vi "Send-clients-list.vi"(8 "error in (no error)":errorcluster, 9 "Sender ID":i32, 10 "Sender":string, 11 "ModComm in":T1) -> (0 "error out":errorcluster, 3 "ModComm out":T1)   [LabVIEW 2013, in "SLMServer.lvlib" / "SLMServer.lvclass"]
uses:
  SLMServer.lvclass
  Object-reference.ctl
  SA-SLMAPI/Sources/Get-clients/Get-clients.lvclass
  SLMServer.lvclass/SLMServer.ctl
  SA-SLMAPI/Sources/Get-clients/Get-clients.lvclass/Get-clients.ctl
  Read Client IDs.vi
  Read Clients.vi
  SA-SLMAPI/Sources/Get-clients/Write Client IDs.vi
  SA-SLMAPI/Sources/Get-clients/Write Client types.vi
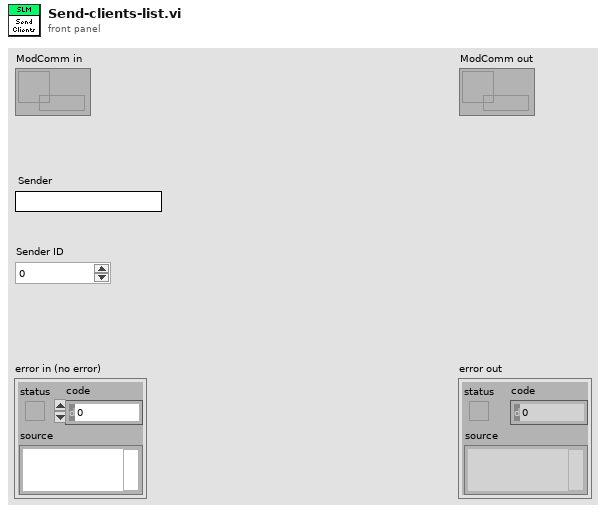
[diagram p1: front panel]
types:
  T1 = typedef "SLMServer.lvlib/SLMServer.lvclass/Object-reference.ctl" = refnum<data-value>
  T2 = typedef "SLMServer.lvlib/SLMServer.lvclass/Supported-module-types.ctl" = enum16{"SLMControl", "PowderDeposition", "CameraVision", "Server", "All", "StrategyParser", "MaterialCharacterization", "StatusMonitor", "SLMSimulation", "LaserCharacterization"}
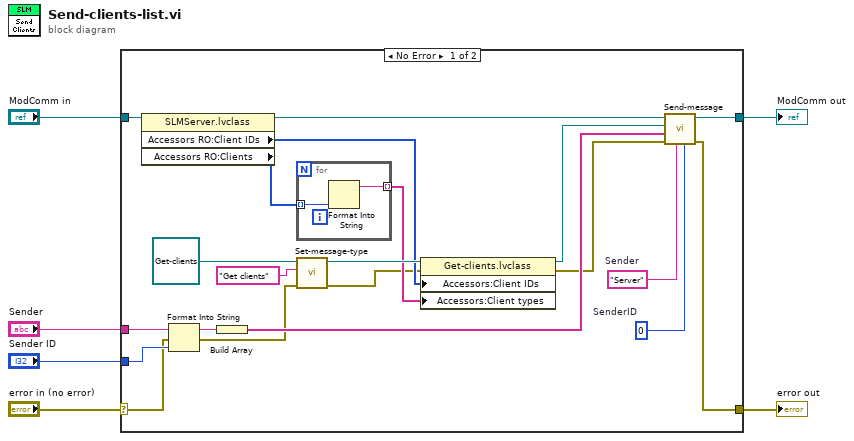
[diagram p0: block diagram]
diagram:
  n1 = case shown="No Error" "error in (no error)" {
    selector: "error in (no error)" -> [w21 w31]
    tunnel: [w7 w31] -> w5
    tunnel: [w26 w30] -> w3
    tunnel: "ModComm in" -> [w27 w30]
    tunnel: "Sender" -> [w23 _]
    tunnel: "Sender ID" -> [w22 _]
    frame No Error {
      w24 = 0  # SenderID
      w25 = "Server"  # Sender
      n2 = property class="SLMServer.lvclass"(reference=w27) -> (reference out=w18:T1, "Accessors RO:Client IDs"=w13:i32[], "Accessors RO:Clients"=w15:T2[])  [unwired: 1 in, 1 out]
      n3 = Format Into String(initial string=w23, error in=w21, w22) -> (resulting string=w20:string, error out=w8:errorcluster)  [unwired: 1 in]
      n4 = Build Array(w20) -> (w19:string[])
      n5 = for {
        tunnel: w15 -> [w29] mode=indexing
        tunnel: [w28] -> w12 mode=indexing
        n6 = Format Into String(w29) -> (resulting string=w28:string)  [unwired: 3 in, 1 out]
      }
      n7 = call-dynamic "Set-message-type.vi"("error in (no error)"=w8, "Message type"="Get clients", "Message in"=refnum<class "Get-clients.lvclass"> refnum ("Module-communication.lvlib:Get-clients.lvclass")) -> ("error out"=w10:errorcluster, "Message out"=w14:refnum<class "Get-clients.lvclass">)  [unwired: 7 in]
      n8 = property class="Get-clients.lvclass"(reference=w14, error in=w10, "Accessors:Client IDs"=w13, "Accessors:Client types"=w12) -> (reference out=w11:refnum<class "Get-clients.lvclass">, error out=w9:errorcluster)
      n9 = call "Send-message.vi"("SenderID"=w24, "Sender"=w25, "error in (no error)"=w9, "Receivers"=w19, "Message"=w11, "Server in"=w18) -> ("error out"=w7:errorcluster, "Server out"=w26:T1)  [unwired: 4 in]
    }
    frame Error {
    }
  }
  "error out" <- w5
  "ModComm out" <- w3
